vi "Apply cool-down delay.vi"(8 "error in (no error)":errorcluster, 11 "Logging queue element in":T1 {"Ref Dwell time (us)" format="%#.6g"; "Frame Size" items=["100X100"=100, "128X128"=128, "200X200"=200, "256X256"=256, "512X512"=512, "1024x1024"=1024, "2048x2048"=2048]; "Dwell time (us)" format="%#.6g"}) -> (0 "error out":errorcluster)   [LabVIEW 2017]
uses:
  Typedefs/Logging queue element.ctl
  Typedefs/Imaging Protocols enum.ctl
  Typedefs/Frame Size.ctl
  Typedefs/Acquired points count.ctl
  Global Variables/General Globals.vi
  Global Variables/gl_UI Ctrl Refs.vi
panel:
  in  "milliseconds to wait":u32
  in  "(-) Offset (sec)":dbl=0.0013 format="%#_13g"
  # "<--- fine-tuning"
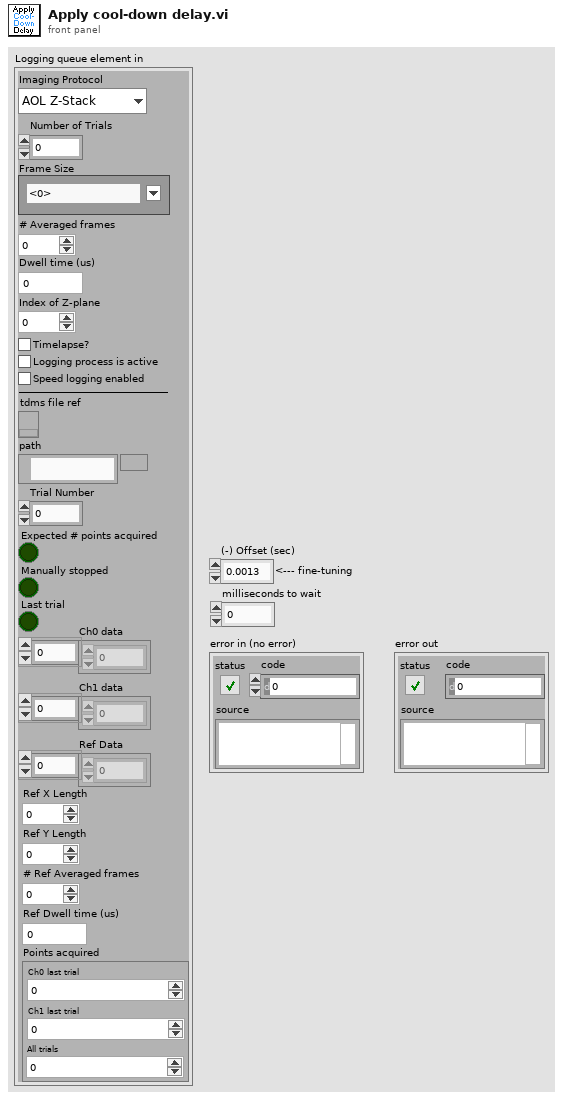
[diagram p1: front panel]
types:
  T1 = typedef "Logging queue element.ctl" = cluster{"Imaging Protocol":T2, "Number of Trials":u16, "Frame Size":T3, "# Averaged frames":u16, "Dwell time (us)":dbl, "Index of Z-plane":i32, "Timelapse?":bool, "Logging process is active":bool, "Speed logging enabled":bool, "tdms file ref":refnum<k34>, "path":path, "Trial Number":i32, "Expected # points acquired":bool, "Manually stopped":bool, "Ch0 data":u32[], "Ch1 data":u32[], "Ref Data":u32[], "Last trial":bool, "Ref Dwell time (us)":dbl, "# Ref Averaged frames":u16, "Ref X Length":u16, "Ref Y Length":u16, "Points acquired":T4}
  T2 = typedef "Imaging Protocols enum.ctl" = enum16{"AOL Z-Stack", "Motor Z Stack", "Functional Acquisition", "Single Plane Acquisition", "Volume Acquisition", "Live Imaging", "Live Plane Imaging", "Live Volume Imaging"}
  T3 = typedef "Frame Size.ctl" = u16
  T4 = typedef "Acquired points count.ctl" = cluster{"Ch0 last trial":u64, "Ch1 last trial":u64, "All trials":u64}
  T5 = typedef "UI ctrl refs cluster.ctl" = cluster{"Top level VI path":path, "Top level VI ref":refnum<vi>, "User menu ref":refnum<k9>, "Sub Panel control":refnum<vi>, "Imaging Param Tab":refnum<vi>, "Occurrence-Start drivers":refnum<k4>, "Occurrence-Speed logging initialised":refnum<k4>, "Occurrence-XYZ stage initialised":refnum<k4>, "Exit button":refnum<vi>, "Status ind":refnum<vi>, "Set as origin":refnum<vi>, "Speed Logging":refnum<vi>, "Time Lapse":refnum<vi>, "Live Imaging":refnum<vi>, "AOL Z Stack":refnum<vi>, "Motor Z Stack":refnum<vi>, "Funct Acq button":refnum<vi>, "Hard Shutter":refnum<vi>, "Virtual Shutter":refnum<vi>, "Laser Power":refnum<vi>, "AOL Mode":refnum<vi>, "Frame Size":refnum<vi>, "Field of View":refnum<vi>, "Dwell Time":refnum<vi>, "Zoom":refnum<vi>, "AOL Z":refnum<vi>, "Objective":refnum<vi>, "Axis":refnum<vi>, "Paths & Names":refnum<vi>, "Experiment folder path (ind.)":refnum<vi>, "Last State (Ind.)":refnum<vi>, "Laser wavelength ind (nm)":refnum<vi>, "Averages":refnum<vi>, "Angle (degrees)":refnum<vi>, "X centre":refnum<vi>, "Y centre":refnum<vi>, "Plane Mode":refnum<vi>, "# Planes":refnum<vi>, "Z Start":refnum<vi>, "Z Stop":refnum<vi>, "Z Step":refnum<vi>, "PMT 1":refnum<vi>, "PMT 2":refnum<vi>, "Stage XYZ Position":refnum<vi>, "Pockels@Z Start":refnum<vi>, "Pockels@Z Stop":refnum<vi>, "Obtain Z Start":refnum<vi>, "Obtain Z Stop":refnum<vi>, "Live stim.trig.period":refnum<vi>, "Live stim.trig.enable":refnum<vi>, "Movement Correction":refnum<vi>, "Load Reference Image":refnum<vi>, "XY Stage Move":refnum<vi>, "MovCor Cluster":refnum<vi>, "RefDAQParam":refnum<vi>, "Funct. Acq. Pockels Modulation":refnum<vi>, "Background MovCor":refnum<vi>, "Ref Laser Power":refnum<vi>, "Enable Video Recording":refnum<vi>, "Video Record-Live Imaging":refnum<vi>, "Video Record-Funct acq":refnum<vi>, "Reference Source":refnum<vi>, "AOL Z-stack Chirps Ready (ind)":refnum<vi>, "Target time between mov.cor. ref triggers (ms)":refnum<vi>, "Funct. Acq. Ref frame save":refnum<vi>, "Tracking button":refnum<vi>, "Show ref plots window":refnum<vi>, "Center freq ind (nm)":refnum<vi>, "Pickup mode (ind)":refnum<vi>, "Logging queue (ind)":refnum<vi>, "Back aperture power (ind.)":refnum<vi>, "Power after objective (ind.)":refnum<vi>, "Switch user":refnum<vi>}
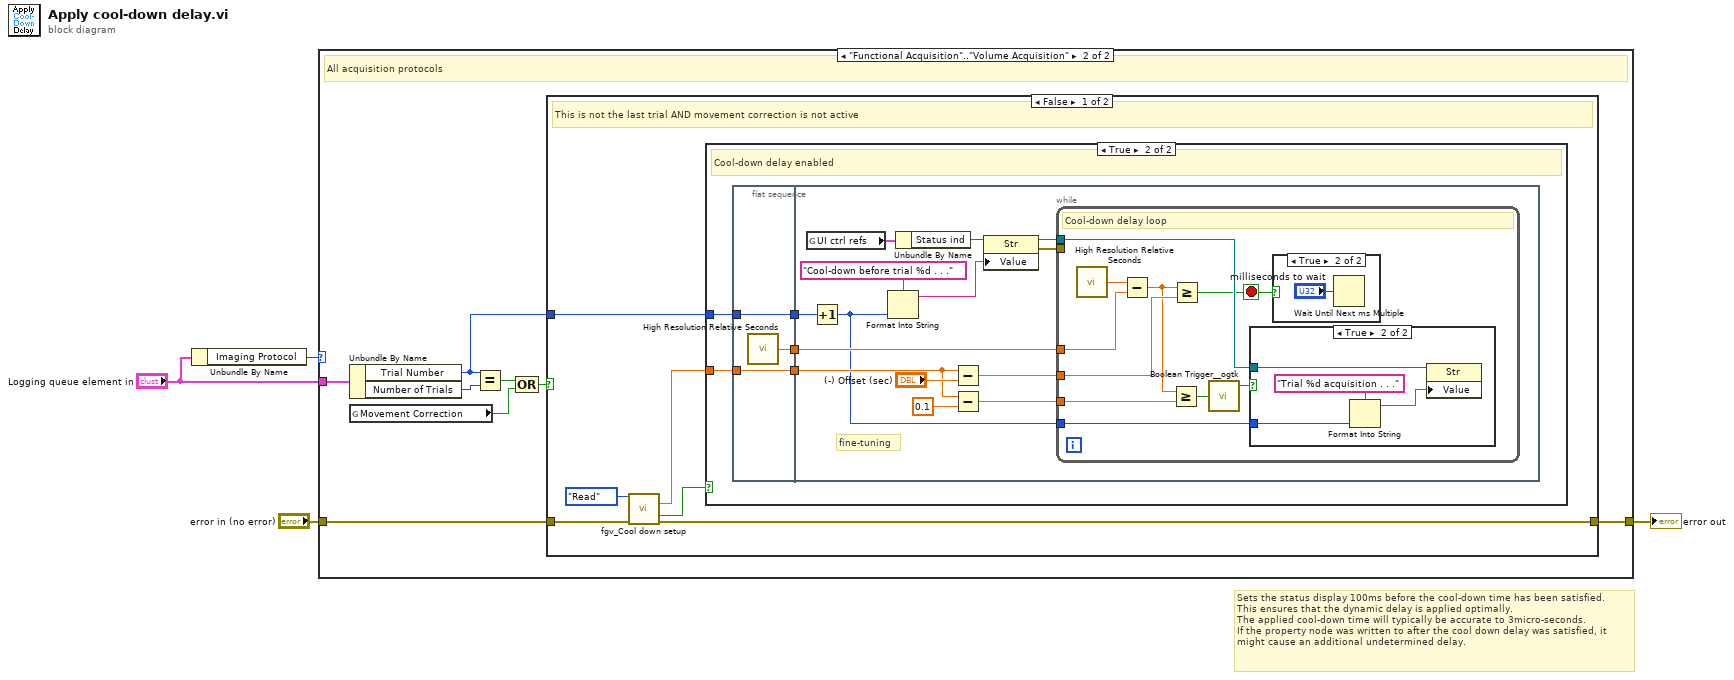
[diagram p0: block diagram]
diagram:
  # "Sets the status display 100ms before the cool-down time has been satisfied.\nThis ensures that the dynamic delay is applied optimally.\nThe applied cool-down time will typically be accurate to 3micro-seconds.\nIf the property node was written to after the cool down delay was satisfied, it might cause an additional undetermined delay."
  n1 = Unbundle By Name("Logging queue element in") -> ("Imaging Protocol"=w2:T2)
  n2 = case shown="\"Functional Acquisition\"..\"Volume Acquisition\"" w2 {
    tunnel: [w5 w13] -> w4
    tunnel: "error in (no error)" -> [w5 w12]
    tunnel: "Logging queue element in" -> [_ w11]
    frame Default {
      # "All other protocols"
    }
    frame "Functional Acquisition".."Volume Acquisition" {
      # "All acquisition protocols"
      n3 = Unbundle By Name(w11) -> ("Trial Number"=w9:i32, "Number of Trials"=w10:u16)
      n4 = global read "General Globals.vi" "Movement Correction"() -> (w7:bool)
      n5 = Equal?(x=w9, y=w10) -> (x = y?=w8:bool)
      n6 = Compound Arithmetic op=OR(w8, w7) -> (w6:bool)
      n7 = case shown="False" w6 {
        tunnel: [w19 w57] -> w13
        tunnel: w12 -> [w18 w57]
        tunnel: w9 -> [w14 _]
        frame False {
          # "This is not the last trial AND movement correction is not active"
          n8 = call "fgv_Cool down setup.vi"("Function"=enum16{"Intialize", "Write", "Read", "Clear"}."Read", "error in (no error)"=w18) -> ("Cool-down time (s)"=w15:dbl, "Enable cool-down time"=w16:bool, "error out"=w19:errorcluster)  [unwired: 11 in]
          n9 = case shown="True" w16 {
            tunnel: w15 -> [_ w24]
            tunnel: w14 -> [_ w21]
            frame False {
              # "The status indicator is set by the \"Logging module-status updater.vi\""
              # "Cool-down delay disabled"
            }
            frame True {
              # "Cool-down delay enabled"
              n10 = flat-sequence {
                tunnel: w24 -> [w27]
                tunnel: [w27] -> w23
                tunnel: [w26] -> w22
                tunnel: w21 -> [w25]
                tunnel: [w25] -> w20
                tunnel: w23 -> [w30]
                tunnel: w22 -> [w40]
                tunnel: w20 -> [w29]
                frame #0 {
                  n11 = call <vilib>:"High Resolution Relative Seconds.vi"() -> ("relative seconds"=w26:dbl)
                }
                frame #1 {
                  # "fine-tuning"
                  n12 = global read "gl_UI Ctrl Refs.vi" "UI ctrl refs"() -> (w38:T5)
                  n13 = Increment(x=w29) -> (x+1=w28:i32)
                  n14 = Format Into String(format string="Cool-down before trial %d . . ." ("Acquiring and Logging..."), w28) -> (resulting string=w36:string)  [unwired: 2 in, 1 out]
                  n15 = Unbundle By Name(w38) -> ("Status ind"=w37:refnum<vi>)
                  n16 = Subtract(x=w30, y="(-) Offset (sec)") -> (x-y=w34:dbl)
                  n17 = Subtract(x=w30, y=0.1) -> (x-y=w32:dbl)
                  n18 = property class="Str"(reference=w37, "Value"=w36) -> (reference out=w31:refnum<vi>, error out=w35:errorcluster)  [unwired: 1 in]
                  n19 = while {
                    tunnel: w40 -> [w50]
                    tunnel: w34 -> [w49]
                    tunnel: w35 -> [_]
                    tunnel: w32 -> [w47]
                    tunnel: w31 -> [w44]
                    tunnel: w28 -> [w42]
                    stop <- w43 stop-if-true
                    # "Cool-down delay loop"
                    n20 = call <vilib>:"High Resolution Relative Seconds.vi"() -> ("relative seconds"=w51:dbl)
                    n21 = Subtract(x=w51, y=w50) -> (x-y=w48:dbl)
                    n22 = Greater Or Equal?(x=w48, y=w47) -> (x >= y?=w46:bool)
                    n23 = Greater Or Equal?(x=w48, y=w49) -> (x >= y?=w43:bool)
                    n24 = call <userlib>:"Boolean Trigger__ogtk.vi"("Boolean Input"=w46) -> ("Rising Edge"=w45:bool)  [unwired: 1 in, 1 out]
                    n25 = case shown="True" w45 {
                      tunnel: w44 -> [_ w55]
                      tunnel: w42 -> [_ w52]
                      frame False {
                      }
                      frame True {
                        n26 = Format Into String(format string="Trial %d acquisition . . ." ("Acquiring and Logging..."), w52) -> (resulting string=w53:string)  [unwired: 2 in, 1 out]
                        n27 = property class="Str"(reference=w55, "Value"=w53) -> ()  [unwired: 1 in, 2 out]
                      }
                    }
                    n28 = case shown="True" w43 {
                      frame False {
                      }
                      frame True {
                        n29 = Wait Until Next ms Multiple(millisecond multiple="milliseconds to wait") -> ()  [unwired: 1 out]
                      }
                    }
                  }
                }
              }
            }
          }
        }
        frame True {
          # "Last trial OR Movement correction is active"
        }
      }
    }
  }
  "error out" <- w4
